vi "RSZVB Set External Signal Generator Output.vi"(8 "error in (no error)":errorcluster {"code" format="%.0x"}, 9 "Ext Signal Generator Output (Off)":bool, 10 "Channel (1)":i32=1, 11 "VISA session":refnum<visa-resource-name>) -> (0 "error out":errorcluster {"code" format="%.0x"}, 3 "dup VISA session":refnum<visa-resource-name>)   [LabVIEW 2011]
doc: "This VI routes either the R&S ZVA pulse generator signals or the external pulse generator signals to the PULSE GENERATOR OUT connector.\n\nRemote-control command(s):\n[SENSe<Ch>:]EUNit:PGENerator:OUTPut:EXTernal"
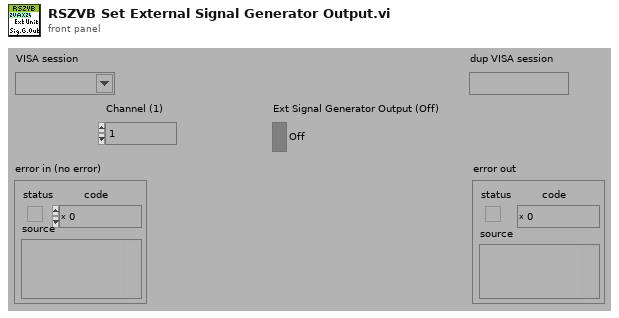
[diagram p1: front panel]
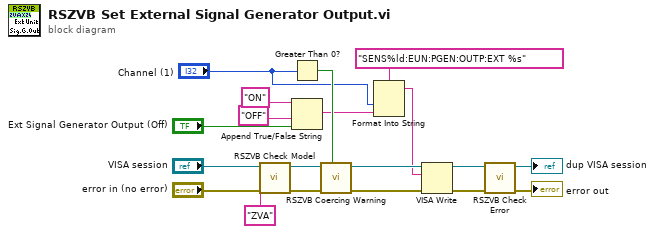
[diagram p0: block diagram]
diagram:
  n1 = call "RSZVB Check Model.vi"("error in (no error)"="error in (no error)", "Model"="ZVA" ("Options"), "VISA session"="VISA session") -> ("error out"=w7:errorcluster, "dup VISA session"=w8:refnum<visa-resource-name>)  [unwired: 7 in]
  n2 = Greater Than 0?(x="Channel (1)") -> (x > 0?=w13:bool)
  n3 = Append True/False String(1:"Ext Signal Generator Output (Off)", 2:"OFF", 3:"ON") -> (0:w10:string)  [unwired: 1 in]
  n4 = call "RSZVB Coercing Warning.vi"("In Range?"=w13, "error in (no error)"=w7, "VISA session"=w8) -> ("error out"=w17:errorcluster, "dup VISA session"=w18:refnum<visa-resource-name>)  [unwired: 7 in]
  n5 = Format Into String(format string="SENS%ld:EUN:PGEN:OUTP:EXT %s", "Channel (1)", w10) -> (resulting string=w14:string)  [unwired: 2 in, 1 out]
  n6 = VISA Write(VISA resource name=w18, write buffer=w14, error in (no error)=w17) -> (VISA resource name out=w15:refnum<visa-resource-name>, error out=w16:errorcluster)  [unwired: 1 out]
  n7 = call "RSZVB Check Error.vi"("error in (no error)"=w16, "VISA session"=w15) -> ("error out"=→"error out":errorcluster, "dup VISA session"=→"dup VISA session":refnum<visa-resource-name>)  [unwired: 8 in]
